vi "Autosetup.vi"(8 "error in (no error)":errorcluster, 11 "VISA resource name":refnum<visa-resource-name>) -> (0 "error out":errorcluster, 3 "VISA resource name out":refnum<visa-resource-name>)   [LabVIEW 2020, in "Agilent 90000 Series.lvlib"]
doc: "Causes the oscilloscope to evaluate all input waveforms and find the optimum conditions for displaying the waveform."
uses:
  Agilent 90000 Series.lvlib
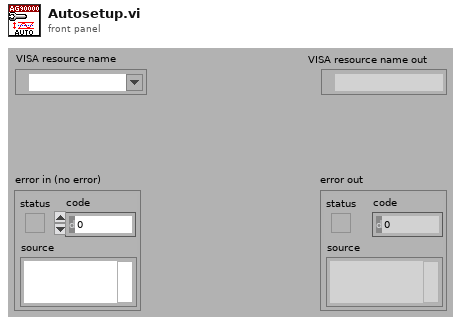
[diagram p1: front panel]
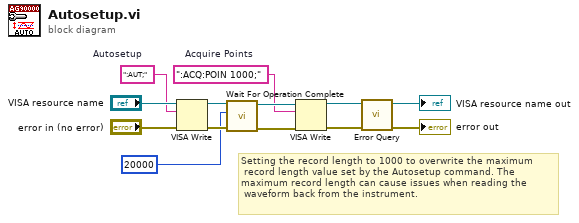
[diagram p0: block diagram]
diagram:
  w2 = ":ACQ:POIN 1000;"  # Acquire Points
  w11 = ":AUT;"  # Autosetup
  # "Setting the record length to 1000 to overwrite the maximum\n record length value set by the Autosetup command. The \nmaximum record length can cause issues when reading the\n waveform back from the instrument."
  n1 = VISA Write(VISA resource name="VISA resource name", write buffer=w11, error in (no error)="error in (no error)") -> (VISA resource name out=w8:refnum<visa-resource-name>, error out=w7:errorcluster)  [unwired: 1 out]
  n2 = call "Wait For Operation Complete.vi"("error in (no error)"=w7, "Maximum Time (5000ms)"=u32 20000, "VISA resource name"=w8) -> ("error out"=w5:errorcluster, "VISA resource name out"=w6:refnum<visa-resource-name>)  [unwired: 7 out]
  n3 = VISA Write(VISA resource name=w6, write buffer=w2, error in (no error)=w5) -> (VISA resource name out=w3:refnum<visa-resource-name>, error out=w4:errorcluster)  [unwired: 1 out]
  n4 = call "Error Query.vi"("error in (no error)"=w4, "VISA resource name"=w3) -> ("error out"=→"error out":errorcluster, "VISA resource name out"=→"VISA resource name out":refnum<visa-resource-name>)  [unwired: 8 out]
